vi "Case selector test.vi"() -> ()   [LabVIEW 2013]
panel:
  out "String":string
  in  "stop":bool
  in  "Enum":enum16{"Option 1", "Option 2", "Option 3"}(ring)
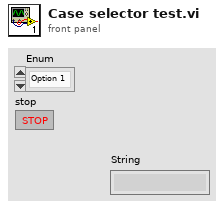
[diagram p1: front panel]
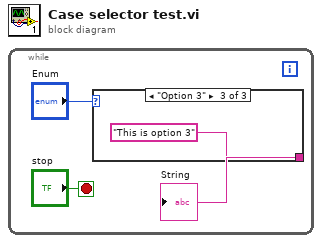
[diagram p0: block diagram]
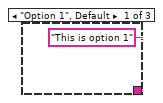
[diagram p2: hidden frame]
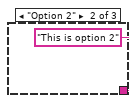
[diagram p3: hidden frame]
diagram:
  n1 = while {
    stop <- "stop" stop-if-true
    n2 = case shown="\"Option 3\"" "Enum" {
      tunnel: ["This is option 1" "This is option 2" "This is option 3"] -> w2
      frame "Option 1", Default {
      }
      frame "Option 2" {
      }
      frame "Option 3" {
      }
    }
    "String" <- w2
  }
